vi "message service.vi"(8 "error in":errorcluster, 10 "response queue":T1, 11 "command queue":T1) -> (0 "error out":errorcluster)   [LabVIEW 2013, in "TBD execution service.lvlib"]
doc: "This VI contains a queued message handler process with an associated message API that allows a user to load up a configuration file, launch the configuration, and communicate with the engines contained in that configuration. \n\nThis process can be useful when you want to support the control of this target by one or more connected hosts. It also allows users to change configuration files without rebooting the target."
uses:
  TBD execution service.lvlib
  <vilib>/NI/AMC/Message Queue.ctl
  <vilib>/NI/AMC/Message.ctl
  <vilib>/NI/Tools/Keyed Array/KeyedArray.ctl
  <vilib>/NI/Configuration Framework/class discovery singleton/class discovery singleton methods.ctl
  SubVIs/configuration elements.ctl
  <vilib>/NI/Tag Bus Data Framework/Framework Configuration Classes/platypus configuration/engines cluster.ctl
  <vilib>/NI/Module Execution Interface/Engine Configuration/engine configuration.lvclass
  <vilib>/NI/Tag Bus Module Framework/module configuration/TBM module configuration.lvclass
  <vilib>/NI/Module Execution Interface/Engine Runtime/Engine Runtime Interface.lvclass
  <vilib>/NI/Tag Bus Module Framework/runtime/TBM module execution interface.lvclass
  <vilib>/NI/Tag Bus Data Framework/Framework Configuration Classes/target runtime/PL_Target Runtime.lvclass
  SubVIs/engine status data.ctl
  <vilib>/NI/Module Execution Interface/Engine Runtime/Execution States.ctl
  <vilib>/NI/Module Execution Interface/Engine Runtime/Fault.ctl
  <vilib>/NI/Tag Bus Module Framework/runtime/error classification.ctl
  <vilib>/NI/AMC/Read Termination Message.vi
  <vilib>/NI/AMC/Create Single Message.vi
  <vilib>/NI/AMC/Globals.vi
  <vilib>/NI/Configuration Framework/class discovery singleton/class discovery singleton.lvlib
  <vilib>/NI/AMC/AMC.lvlib
  <vilib>/NI/Tag Bus Module Framework/FPGA manager/methods.ctl
  <vilib>/NI/Tag Bus Module Framework/FPGA manager/FPGA manager.lvlib
  <vilib>/userdefined/High Color/nirio_resource_hc.ctl
  <vilib>/rvi/interface/nirviOpenFPGA/nirviOpenFPGA.xnode
  <vilib>/NI/Tag Bus Data Framework/Framework Configuration Classes/platypus configuration/PLConfigurationSerializer.lvlib
  <vilib>/NI/Configuration Framework/tree serializer/NISE_CEF_TreeSerializer.lvlib
  <vilib>/NI/Tag Bus Data Framework/Framework Configuration Classes/flattened data interface/PL_Serialization Interface.lvlib
  <vilib>/NI/Tools/Keyed Array/Tools_KeyedArray.lvlib
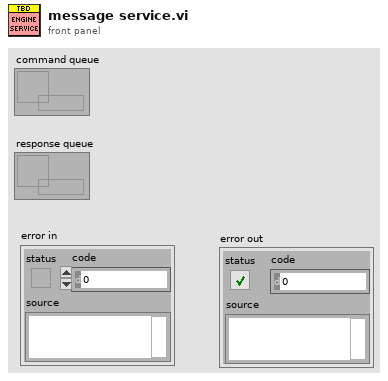
[diagram p1: front panel]
types:
  T1 = typedef "AMC.lvlib/Message Queue.ctl" = refnum<queue>
  T2 = typedef "class discovery singleton.lvlib/class discovery singleton methods.ctl" = enum16{"add search paths", "load class by name", "list available classes", "get class path"}
  T3 = typedef "nirio_resource_hc.ctl" = tag
  T4 = typedef "FPGA manager.lvlib/methods.ctl" = enum16{"initialize bitfile", "cache bitfile", "locate bitfile", "close bitfile"}
  T5 = typedef "TBD execution service.lvlib/configuration elements.ctl" = cluster{"Name":string, "opened?":bool, "configuration":T6, "engine":refnum<class "Engine Runtime Interface.lvclass">, "modules":refnum<class "TBM module execution interface.lvclass">[]}
  T6 = typedef "PLConfigurationSerializer.lvlib/engines cluster.ctl" = cluster{"engine configuration":refnum<class "engine configuration.lvclass">, "modules":refnum<class "TBM module configuration.lvclass">[]}
  T7 = typedef "TBD execution service.lvlib/engine status data.ctl" = cluster{"Name":string, "Engine State":T8, "Faults":T9[], "Engine Error":errorcluster}
  T8 = typedef "Engine Runtime Interface.lvclass/Execution States.ctl" = enum16{"Init", "Pre-Operational", "Safe-Operational", "Operational", "Stopped"}
  T9 = typedef "Engine Runtime Interface.lvclass/Fault.ctl" = cluster{"code":i32, "error classification":T10, "Source GUID":string, "first reported time":timestamp, "number reported":u32, "last reported time":timestamp}
  T10 = typedef "TBM module execution interface.lvclass/error classification.ctl" = enum16{"unknown", "none", "trivial", "recoverable", "critical"}
  T11 = typedef "TBD execution service.lvlib/command commands to rtexe process.ctl" = enum16{"Initialize", "Add Search Paths", "Load from File", "Unload File", "Open All Engines", "Open Single Engine", "Initialize All Engines", "Initialize Single Engine", "Start All", "Start Single", "Pause All", "Pause Single", "Stop All", "Stop Single", "Close All", "Close Single", "Set Safe State All", "Set Safe State Single", "Get Status", "Exit", "Error", "Load Bitfile", "Unload Bitfile", "Clear Faults Single", "Clear Faults All"}
  T12 = typedef "NISE_CEF_TreeSerializer.lvlib/base file format.ctl" = cluster{"version":string, "data":string}
  T13 = typedef "NISE_CEF_TreeSerializer.lvlib/flat hierarchy.ctl" = cluster{"hierarchy structure":T14, "instance data":T16[]}
  T14 = typedef "NISE_CEF_TreeSerializer.lvlib/full hierarchy.ctl" = cluster{"root":string, "hierarchy":T15[]}
  T15 = typedef "NISE_CEF_TreeSerializer.lvlib/hierarchy element.ctl" = cluster{"current node":string, "children":string[]}
  T16 = typedef "NISE_CEF_TreeSerializer.lvlib/instance data.ctl" = cluster{"ID":string, "Alias":string, "class":string, "version":string, "data":string}
  T17 = typedef "PLConfigurationSerializer.lvlib/targets cluster.ctl" = cluster{"Target Configuration":refnum<class "PL_Target Configuration.lvclass">, "engines":T6[]}
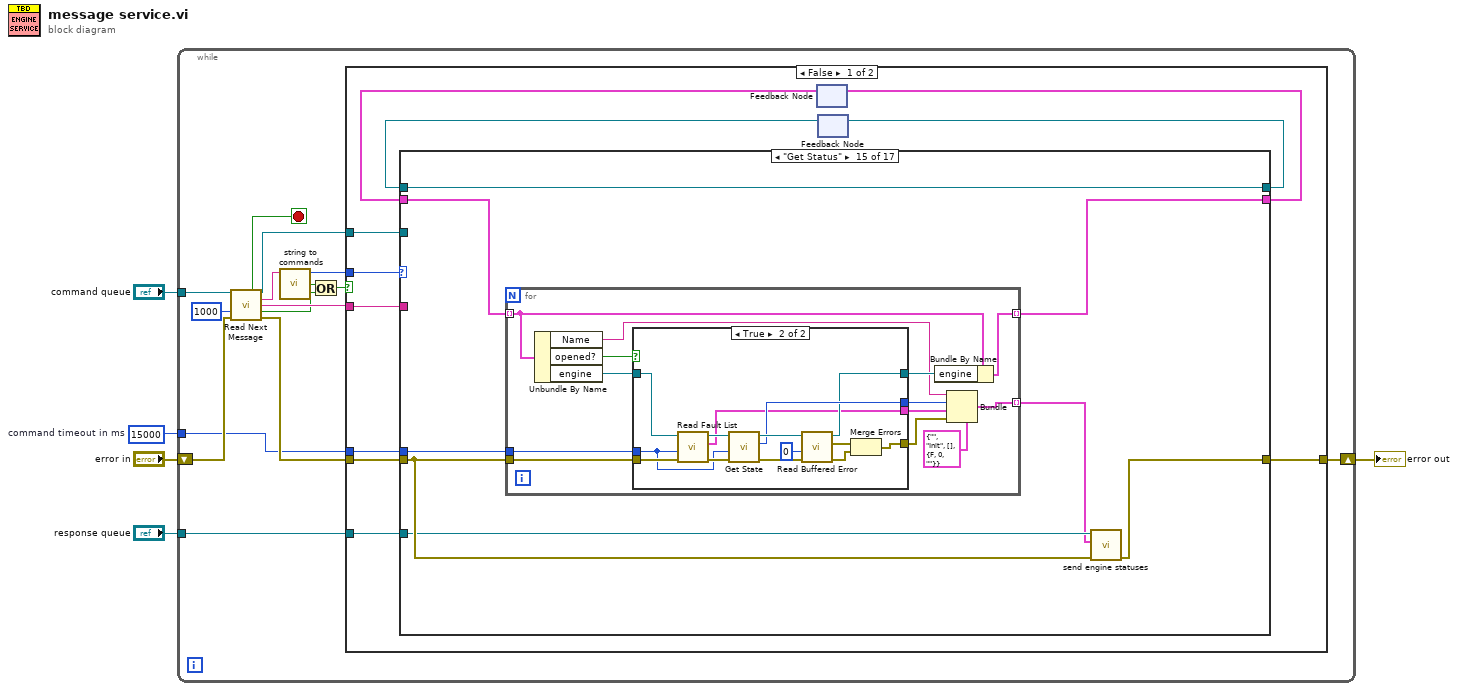
[diagram p0: block diagram]
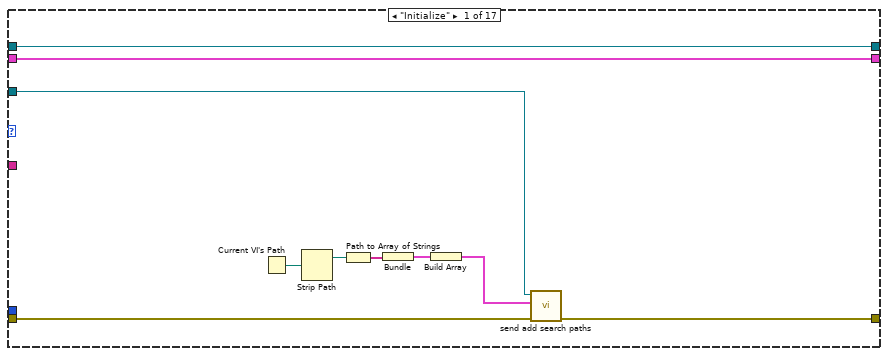
[diagram p2: hidden frame]
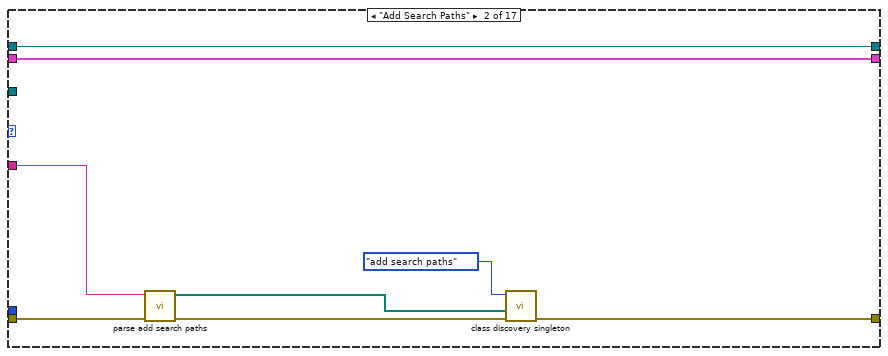
[diagram p3: hidden frame]
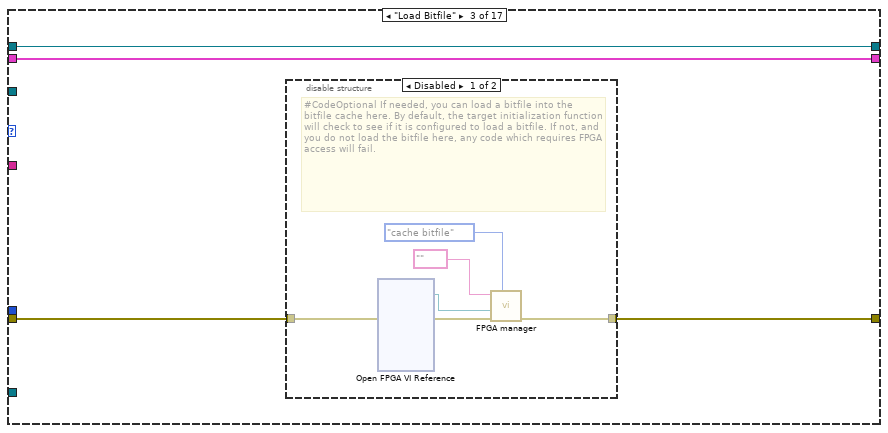
[diagram p4: hidden frame]
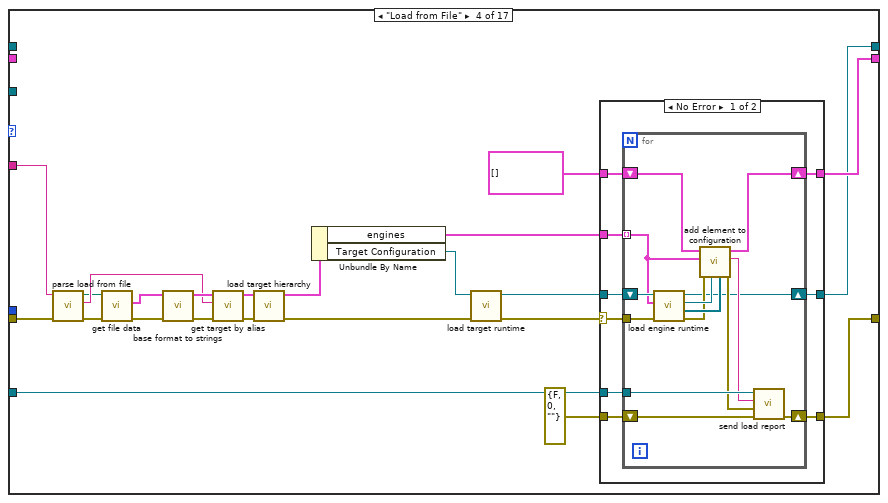
[diagram p6: hidden frame]
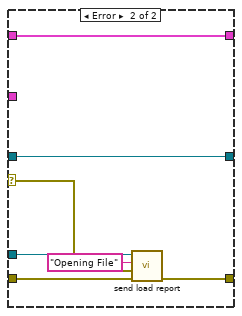
[diagram p7: hidden frame]
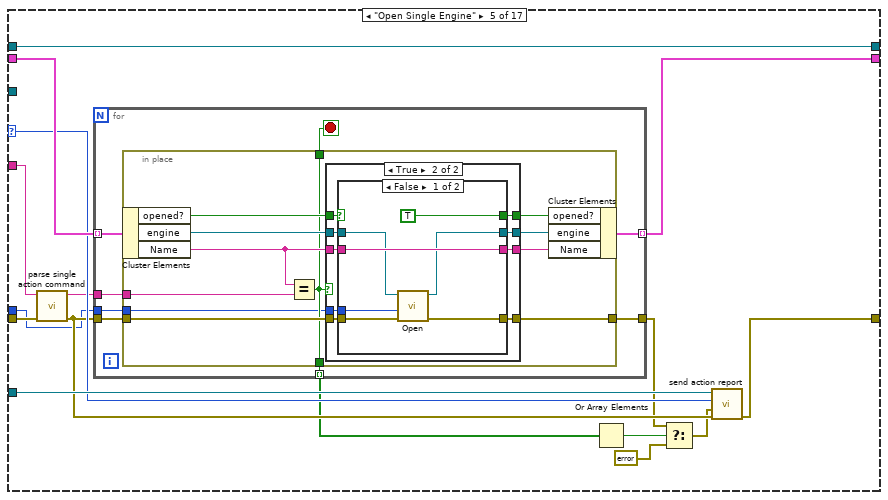
[diagram p8: hidden frame]
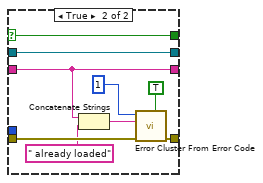
[diagram p10: hidden frame]
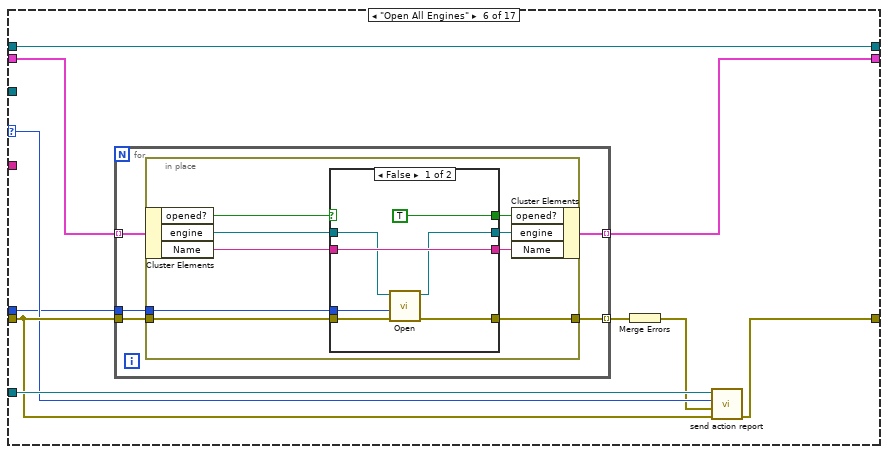
[diagram p11: hidden frame]
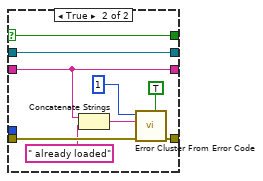
[diagram p12: hidden frame]
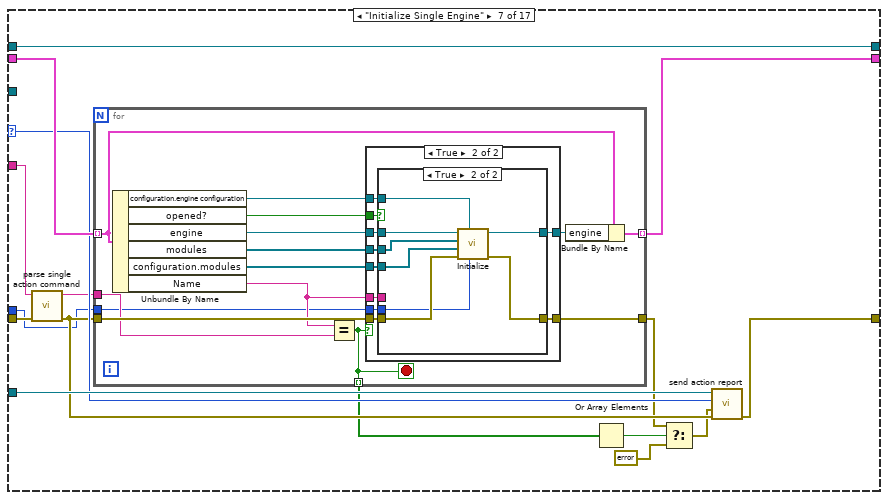
[diagram p13: hidden frame]
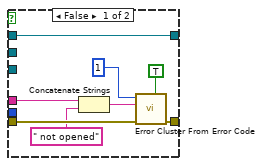
[diagram p15: hidden frame]
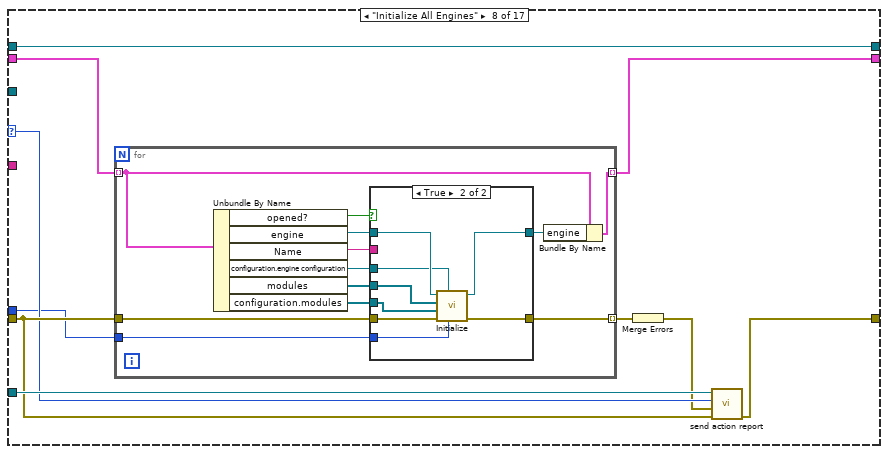
[diagram p16: hidden frame]
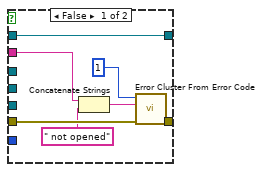
[diagram p17: hidden frame]
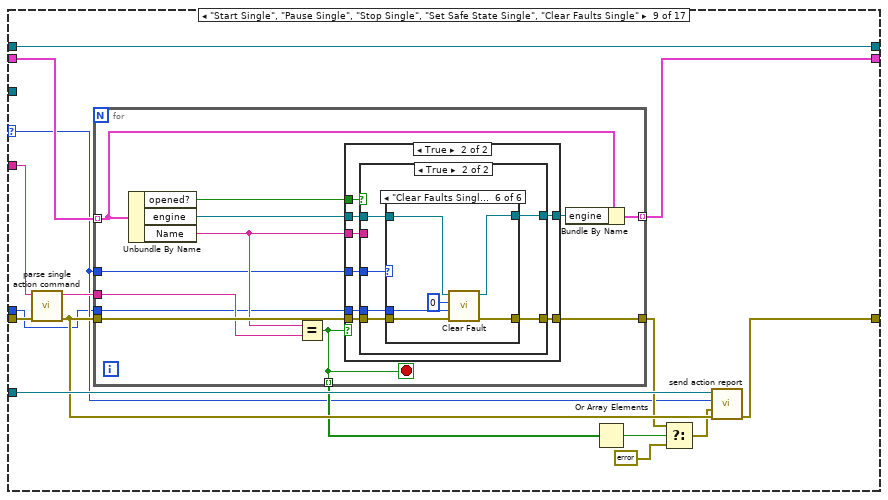
[diagram p18: hidden frame]
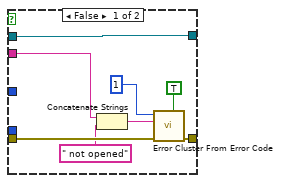
[diagram p20: hidden frame]
diagram:
  w1 = 15000  # command timeout in ms
  n1 = while {
    tunnel: "command queue" -> [w18]
    shift-right: [w20] -> w2
    shift-left: "error in" -> [w15]
    tunnel: "response queue" -> [w19]
    tunnel: w1 -> [w6]
    stop <- w17 stop-if-true
    n2 = call <vilib>:"Read Next Message.vi"("message queue in"=w18, "timeout (1 ms)"=1000, "error in"=w15) -> ("exit process?"=w17:bool, "message queue out"=w7:T1, "message name"=w12:string, "message value"=w16:string, "timed out?"=w10:bool, "error out"=w14:errorcluster)  [unwired: 5 in, 2 out]
    n3 = call "string to commands.vi"("command string"=w12) -> ("invalid"=w11:bool, "commands"=w8:T11)  [unwired: 9 in]
    n4 = Or(x=w11, y=w10) -> (x .or. y?=w9:bool)
    n5 = case shown="False" w9 {
      tunnel: w16 -> [w31 _]
      tunnel: [w30 w654] -> w20
      tunnel: w19 -> [w29 _]
      tunnel: w14 -> [w28 w654]
      tunnel: w8 -> [w27 _]
      tunnel: w7 -> [w26 _]
      tunnel: w6 -> [w21 _]
      frame False {
        n6 = feedback #1() -> (w24:T5[])  [unwired: 1 in]
        n7 = feedback #2() -> (w22:refnum<class "PL_Target Runtime.lvclass">)  [unwired: 1 in]
        n8 = case shown="\"Get Status\"" w27 {
          selector: w27 -> [_ _ _ _ w125 w181 w229 w279 w315 w398 w471 w526 _ _ _ _ w623]
          tunnel: w31 -> [_ w43 _ w83 w122 _ w226 _ w322 _ w468 _ _ _ _ _ _]
          tunnel: [w41 w49 w53 w81 w128 w186 w232 w284 w327 w404 w474 w531 w565 w569 w581 w617 w628] -> w25
          tunnel: w24 -> [w41 w49 w53 _ w129 w187 w233 w285 w328 w405 w475 w532 w565 w569 w582 w617 w629]
          tunnel: [w39 w47 w51 w80 w126 w183 w230 w281 w325 w401 w472 w528 w562 w567 w579 w614 w626] -> w30
          tunnel: w28 -> [w40 w46 w52 w82 w124 w184 w228 w282 w324 w402 w470 w529 w563 w568 w580 w615 w625]
          tunnel: w29 -> [_ _ _ w79 w127 w185 w231 w283 w326 w403 w473 w530 _ _ w578 w613 w624]
          tunnel: w26 -> [w38 _ _ _ _ _ _ _ _ _ _ _ _ _ _ _ _]
          tunnel: [w32 w42 w50 w63 w115 w179 w219 w277 w314 w397 w461 w524 _ w566 w576 w612 w622] -> w23
          tunnel: w22 -> [w32 w42 w50 _ w115 w179 w219 w277 w314 w397 w461 w524 w564 w566 w576 w612 w622]
          tunnel: w21 -> [_ _ _ _ w114 w178 w218 w276 w313 w396 w460 w523 _ _ w575 _ w621]
          frame "Initialize" {
            n9 = Current VI's Path() -> (path=w37:path)
            n10 = Strip Path(path=w37) -> (stripped path=w36:path)  [unwired: 1 out]
            n11 = Path to Array of Strings(0:w36) -> (2:w35:string[])  [unwired: 1 out]
            n12 = Bundle("array of strings"=w35) -> (w34:cluster{"array of strings":string[]})  [unwired: 1 in]
            n13 = Build Array(w34) -> (w33:cluster{"array of strings":string[]}[])
            n14 = call "send add search paths.vi"("error in"=w40, "search paths"=w33, "message queue in"=w38) -> ("error out"=w39:errorcluster)  [unwired: 7 in, 1 out]
          }
          frame "Add Search Paths" {
            n15 = call "parse add search paths.vi"("error in"=w46, "message data"=w43) -> ("error out"=w45:errorcluster, "paths"=w44:path[])  [unwired: 8 in]
            n16 = call <vilib>:"class discovery singleton.vi"("error in"=w45, "Plugin Search Paths"=w44, "method"=class_discovery_singleton_methods."add search paths") -> ("error out"=w47:errorcluster)  [unwired: 5 in, 3 out]
          }
          frame "Load Bitfile" {
            n17 = disable-structure shown="Disabled" {
              disable-tunnel: [w55 w60] -> w51
              disable-tunnel: w52 -> [w54 w60]
              frame Disabled {
                # "#CodeOptional If needed, you can load a bitfile into the bitfile cache here. By default, the target initialization function will check to see if it is configured to load a bitfile. If not, and you do not load the bitfile here, any code which requires FPGA access will fail."
                n18 = xnode "Open FPGA VI Reference"("error in"=w54) -> ("FPGA VI Reference Out"=w58:refnum<k20>, "error out"=w59:errorcluster)  [unwired: 1 in]
                n19 = call <vilib>:"FPGA manager.vi"("action"=methods."cache bitfile", "error in"=w59, "bitfile to cache"=w58, "RIO resource"=T3 "") -> ("error out"=w55:errorcluster)  [unwired: 5 in, 2 out]
              }
              frame Enabled {
              }
            }
          }
          frame "Load from File" {
            n20 = call "parse load from file.vi"("error in"=w82, "message data"=w83) -> ("error out"=w61:errorcluster, "target alias"=w64:string, "path"=w62:path)  [unwired: 7 in]
            n21 = call <vilib>:"get file data.vi"("error in"=w61, "Path"=w62) -> ("error out"=w71:errorcluster, "format"=w72:T12)  [unwired: 8 in]
            n22 = call <vilib>:"base format to strings.vi"("error in"=w71, "format"=w72) -> ("error out"=w66:errorcluster, "data"=w68:T13)  [unwired: 8 in]
            n23 = call <vilib>:"get target by alias.vi"("error in"=w66, "alias"=w64, "system hierarchy"=w68) -> ("error out"=w65:errorcluster, "target hierarchy"=w67:T13)  [unwired: 7 in]
            n24 = call <vilib>:"load target hierarchy.vi"("error in"=w65, "target hierarchy"=w67) -> ("error out"=w69:errorcluster, "targets cluster out"=w70:T17)  [unwired: 8 in]
            n25 = Unbundle By Name(w70) -> ("engines"=w77:T6[], "Target Configuration"=w78:refnum<class "PL_Target Configuration.lvclass">)
            n26 = call <vilib>:"load target runtime.vi"("error in"=w69, "target configuration"=w78) -> ("error out"=w73:errorcluster, "target runtime"=w76:refnum<class "PL_Target Runtime.lvclass">)  [unwired: 8 in]
            n27 = case shown="No Error" w73 {
              selector: w73 -> [w85 w112]
              tunnel: [w92 w113] -> w81
              tunnel: [w91 w110] -> w80
              tunnel: w79 -> [w90 w109]
              tunnel: w77 -> [w89 _]
              tunnel: w76 -> [w88 w107]
              tunnel: errorcluster {"status"=FALSE, "code"=0, "source"=""} ("error out") -> [w87 w111]
              tunnel: T5[] [] ("Configuration out") -> [w86 w113]
              tunnel: [w84 w107] -> w63
              frame No Error {
                n28 = for {
                  shift-right: [w106] -> w92
                  shift-left: w86 -> [w105]
                  shift-right: [w103] -> w91
                  shift-left: w87 -> [w100]
                  tunnel: w90 -> [w104]
                  tunnel: w89 -> [w93] mode=indexing
                  shift-right: [w94] -> w84
                  shift-left: w88 -> [w99]
                  tunnel: w85 -> [w98]
                  n29 = call <vilib>:"load engine runtime.vi"("error in"=w98, "engine configuration in"=w93, "Target Runtime in"=w99) -> ("error out"=w95:errorcluster, "Module Runtime Objects"=w96:refnum<class "TBM module execution interface.lvclass">[], "Engine Runtime Object"=w97:refnum<class "Engine Runtime Interface.lvclass">, "Target Runtime out"=w94:refnum<class "PL_Target Runtime.lvclass">)  [unwired: 5 in]
                  n30 = call "add element to configuration.vi"("Module Runtime Objects"=w96, "Engine Runtime Object"=w97, "error in"=w95, "engine configuration in"=w93, "Configuration in"=w105) -> ("error out"=w101:errorcluster, "engine loaded"=w102:string, "Configuration out"=w106:T5[])  [unwired: 4 in]
                  n31 = call "send load report.vi"("error in"=w100, "load error"=w101, "engine loaded"=w102, "message queue in"=w104) -> ("error out"=w103:errorcluster)  [unwired: 6 in, 1 out]
                }
              }
              frame Error {
                n32 = call "send load report.vi"("error in"=w111, "load error"=w112, "engine loaded"="Opening File", "message queue in"=w109) -> ("error out"=w110:errorcluster)  [unwired: 6 in, 1 out]
              }
            }
          }
          frame "Open Single Engine" {
            n33 = call "parse single action command.vi"("error in"=w124, "message data"=w122) -> ("error out"=w123:errorcluster, "engine name"=w121:string)  [unwired: 8 in]
            n34 = for {
              tunnel: w129 -> [w137] mode=indexing
              tunnel: [w136] -> w128 mode=indexing
              tunnel: w121 -> [w133]
              tunnel: [w132] -> w120 mode=indexing
              tunnel: w123 -> [w135]
              tunnel: [w134] -> w118
              tunnel: w114 -> [w130]
              stop <- w131 stop-if-true
              n35 = in-place {
                in-place-border: w135 -> [w145]
                in-place-border: [w144] -> w134
                in-place-border: w133 -> [w141]
                in-place-border: [w139] -> w132
                in-place-border: [w139] -> w131
                in-place-border: w130 -> [w138]
                n36 = in-place-cluster #3(w137) -> ("opened?"=w148:bool, "engine"=w147:refnum<class "Engine Runtime Interface.lvclass">, "Name"=w140:string)
                n37 = Equal?(x=w140, y=w141) -> (x = y?=w139:bool)
                n38 = case shown="True" w139 {
                  tunnel: w148 -> [w152 w161]
                  tunnel: w147 -> [w151 w160]
                  tunnel: [w151 w159] -> w146
                  tunnel: w145 -> [w149 w158]
                  tunnel: [w149 w157] -> w144
                  tunnel: [w150 w156] -> w143
                  tunnel: [w152 w155] -> w142
                  tunnel: w140 -> [w150 w154]
                  tunnel: w138 -> [_ w153]
                  frame False {
                  }
                  frame True {
                    n39 = case shown="False" w161 {
                      selector: w161 -> [_ w169]
                      tunnel: w160 -> [w165 w177]
                      tunnel: [w164 w177] -> w159
                      tunnel: w158 -> [w168 w176]
                      tunnel: [w167 w175] -> w157
                      tunnel: w154 -> [w166 w170]
                      tunnel: [w166 w170] -> w156
                      tunnel: [TRUE ("opened?") w169] -> w155
                      tunnel: w153 -> [w162 _]
                      frame False {
                        n40 = call-dynamic "Open.vi"("error in"=w168, "timeout (-1)"=w162, "Engine Runtime Interface in"=w165) -> ("error out"=w167:errorcluster, "Engine Runtime Interface out"=w164:refnum<class "Engine Runtime Interface.lvclass">)  [unwired: 7 in]
                      }
                      frame True {
                        n41 = Concatenate Strings(w170, " already loaded" ("string")) -> (w172:string)
                        n42 = call <vilib>:"Error Cluster From Error Code.vi"("is warning? (False)"=TRUE, "error in (no error)"=w176, "error message (\"\")"=w172, "error code (0)"=1) -> ("error out"=w175:errorcluster)  [unwired: 5 in]
                      }
                    }
                  }
                }
                n43 = in-place-cluster #3("opened?"=w142, "engine"=w146, "Name"=w143) -> (w136:T5)
              }
            }
            n44 = Or Array Elements(Boolean array=w120) -> (logical OR=w119:bool)
            n45 = Select(t=w118, s=w119, f=errorcluster {"status"=TRUE, "code"=1, "source"="Not found"}) -> (s? t:f=w117:errorcluster)
            n46 = call "send action report.vi"("error in"=w123, "command error"=w117, "commands"=w125, "message queue in"=w127) -> ("error out"=w126:errorcluster)  [unwired: 6 in, 1 out]
          }
          frame "Open All Engines" {
            n47 = for {
              tunnel: w187 -> [w192] mode=indexing
              tunnel: [w191] -> w186 mode=indexing
              tunnel: w184 -> [w190]
              tunnel: [w189] -> w182 mode=indexing
              tunnel: w178 -> [w188]
              n48 = in-place {
                in-place-border: w190 -> [w198]
                in-place-border: [w197] -> w189
                in-place-border: w188 -> [w193]
                n49 = in-place-cluster #4(w192) -> ("opened?"=w201:bool, "engine"=w200:refnum<class "Engine Runtime Interface.lvclass">, "Name"=w196:string)
                n50 = case shown="False" w201 {
                  selector: w201 -> [_ w209]
                  tunnel: w200 -> [w205 w217]
                  tunnel: [w204 w217] -> w199
                  tunnel: w198 -> [w208 w216]
                  tunnel: [w207 w215] -> w197
                  tunnel: w196 -> [w206 w210]
                  tunnel: [w206 w210] -> w195
                  tunnel: [TRUE ("opened?") w209] -> w194
                  tunnel: w193 -> [w202 _]
                  frame False {
                    n51 = call-dynamic "Open.vi"("error in"=w208, "timeout (-1)"=w202, "Engine Runtime Interface in"=w205) -> ("error out"=w207:errorcluster, "Engine Runtime Interface out"=w204:refnum<class "Engine Runtime Interface.lvclass">)  [unwired: 7 in]
                  }
                  frame True {
                    n52 = Concatenate Strings(w210, " already loaded" ("string")) -> (w212:string)
                    n53 = call <vilib>:"Error Cluster From Error Code.vi"("is warning? (False)"=TRUE, "error in (no error)"=w216, "error message (\"\")"=w212, "error code (0)"=1) -> ("error out"=w215:errorcluster)  [unwired: 5 in]
                  }
                }
                n54 = in-place-cluster #4("opened?"=w194, "engine"=w199, "Name"=w195) -> (w191:T5)
              }
            }
            n55 = Merge Errors(w182) -> (w180:errorcluster)
            n56 = call "send action report.vi"("error in"=w184, "command error"=w180, "commands"=w181, "message queue in"=w185) -> ("error out"=w183:errorcluster)  [unwired: 6 in, 1 out]
          }
          frame "Initialize Single Engine" {
            n57 = call "parse single action command.vi"("error in"=w228, "message data"=w226) -> ("error out"=w227:errorcluster, "engine name"=w225:string)  [unwired: 8 in]
            n58 = for {
              tunnel: w233 -> [w247] mode=indexing
              tunnel: [w246] -> w232 mode=indexing
              tunnel: w225 -> [w243]
              tunnel: [w242] -> w224 mode=indexing
              tunnel: w227 -> [w245]
              tunnel: [w244] -> w222
              tunnel: w218 -> [w234]
              stop <- w242 stop-if-true
              n59 = Unbundle By Name(w247) -> ("configuration.engine configuration"=w235:refnum<class "engine configuration.lvclass">, "opened?"=w241:bool, "engine"=w240:refnum<class "Engine Runtime Interface.lvclass">, "modules"=w236:refnum<class "TBM module execution interface.lvclass">[], "configuration.modules"=w237:refnum<class "TBM module configuration.lvclass">[], "Name"=w238:string)
              n60 = Equal?(x=w238, y=w243) -> (x = y?=w242:bool)
              n61 = case shown="True" w242 {
                tunnel: w241 -> [_ w259]
                tunnel: w240 -> [w249 w258]
                tunnel: [w249 w257] -> w239
                tunnel: w245 -> [w248 w256]
                tunnel: [w248 w255] -> w244
                tunnel: w238 -> [_ w254]
                tunnel: w237 -> [_ w253]
                tunnel: w236 -> [_ w252]
                tunnel: w235 -> [_ w251]
                tunnel: w234 -> [_ w250]
                frame False {
                }
                frame True {
                  n62 = case shown="True" w259 {
                    tunnel: w258 -> [w267 w274]
                    tunnel: [w267 w273] -> w257
                    tunnel: w256 -> [w266 w275]
                    tunnel: [w265 w272] -> w255
                    tunnel: w254 -> [w260 _]
                    tunnel: w253 -> [_ w271]
                    tunnel: w252 -> [_ w270]
                    tunnel: w251 -> [_ w269]
                    tunnel: w250 -> [_ w268]
                    frame False {
                      n63 = Concatenate Strings(w260, " not opened" ("string")) -> (w262:string)
                      n64 = call <vilib>:"Error Cluster From Error Code.vi"("is warning? (False)"=TRUE, "error in (no error)"=w266, "error message (\"\")"=w262, "error code (0)"=1) -> ("error out"=w265:errorcluster)  [unwired: 5 in]
                    }
                    frame True {
                      n65 = call-dynamic "Initialize.vi"("timeout in ms"=w268, "Engine Configuration"=w269, "error in"=w275, "module Configurations"=w271, "modules"=w270, "Engine Runtime Interface in"=w274) -> ("error out"=w272:errorcluster, "Engine Runtime Interface out"=w273:refnum<class "Engine Runtime Interface.lvclass">)  [unwired: 4 in]
                    }
                  }
                }
              }
              n66 = Bundle By Name(cluster=w247, "engine"=w239) -> (w246:T5)
            }
            n67 = Or Array Elements(Boolean array=w224) -> (logical OR=w223:bool)
            n68 = Select(t=w222, s=w223, f=errorcluster {"status"=TRUE, "code"=1, "source"="Not found"}) -> (s? t:f=w221:errorcluster)
            n69 = call "send action report.vi"("error in"=w227, "command error"=w221, "commands"=w229, "message queue in"=w231) -> ("error out"=w230:errorcluster)  [unwired: 6 in, 1 out]
          }
          frame "Initialize All Engines" {
            n70 = for {
              tunnel: w285 -> [w297] mode=indexing
              tunnel: [w296] -> w284 mode=indexing
              tunnel: w282 -> [w295]
              tunnel: [w294] -> w280 mode=indexing
              tunnel: w276 -> [w286]
              n71 = Unbundle By Name(w297) -> ("opened?"=w293:bool, "engine"=w292:refnum<class "Engine Runtime Interface.lvclass">, "Name"=w290:string, "configuration.engine configuration"=w289:refnum<class "engine configuration.lvclass">, "modules"=w288:refnum<class "TBM module execution interface.lvclass">[], "configuration.modules"=w287:refnum<class "TBM module configuration.lvclass">[])
              n72 = case shown="True" w293 {
                tunnel: w292 -> [w304 w309]
                tunnel: [w304 w310] -> w291
                tunnel: w295 -> [w303 w311]
                tunnel: [w302 w312] -> w294
                tunnel: w290 -> [w298 _]
                tunnel: w289 -> [_ w308]
                tunnel: w288 -> [_ w307]
                tunnel: w287 -> [_ w306]
                tunnel: w286 -> [_ w305]
                frame False {
                  n73 = Concatenate Strings(w298, " not opened" ("string")) -> (w300:string)
                  n74 = call <vilib>:"Error Cluster From Error Code.vi"("error in (no error)"=w303, "error message (\"\")"=w300, "error code (0)"=1) -> ("error out"=w302:errorcluster)  [unwired: 6 in]
                }
                frame True {
                  n75 = call-dynamic "Initialize.vi"("timeout in ms"=w305, "Engine Configuration"=w308, "error in"=w311, "module Configurations"=w306, "modules"=w307, "Engine Runtime Interface in"=w309) -> ("error out"=w312:errorcluster, "Engine Runtime Interface out"=w310:refnum<class "Engine Runtime Interface.lvclass">)  [unwired: 4 in]
                }
              }
              n76 = Bundle By Name(cluster=w297, "engine"=w291) -> (w296:T5)
            }
            n77 = Merge Errors(w280) -> (w278:errorcluster)
            n78 = call "send action report.vi"("error in"=w282, "command error"=w278, "commands"=w279, "message queue in"=w283) -> ("error out"=w281:errorcluster)  [unwired: 6 in, 1 out]
          }
          frame "Start Single", "Pause Single", "Stop Single", "Set Safe State Single", "Clear Faults Single" {
            n79 = call "parse single action command.vi"("error in"=w324, "message data"=w322) -> ("error out"=w323:errorcluster, "engine name"=w321:string)  [unwired: 8 in]
            n80 = for {
              tunnel: w328 -> [w340] mode=indexing
              tunnel: [w339] -> w327 mode=indexing
              tunnel: w321 -> [w336]
              tunnel: [w335] -> w320 mode=indexing
              tunnel: w323 -> [w338]
              tunnel: [w337] -> w318
              tunnel: w315 -> [w330]
              tunnel: w313 -> [w329]
              stop <- w335 stop-if-true
              n81 = Unbundle By Name(w340) -> ("opened?"=w334:bool, "engine"=w333:refnum<class "Engine Runtime Interface.lvclass">, "Name"=w331:string)
              n82 = Equal?(x=w331, y=w336) -> (x = y?=w335:bool)
              n83 = case shown="True" w335 {
                tunnel: w334 -> [_ w350]
                tunnel: w333 -> [w342 w349]
                tunnel: [w342 w348] -> w332
                tunnel: w338 -> [w341 w347]
                tunnel: [w341 w346] -> w337
                tunnel: w331 -> [_ w345]
                tunnel: w330 -> [_ w344]
                tunnel: w329 -> [_ w343]
                frame False {
                }
                frame True {
                  n84 = case shown="True" w350 {
                    tunnel: w349 -> [w358 w362]
                    tunnel: [w358 w363] -> w348
                    tunnel: w347 -> [w357 w361]
                    tunnel: [w356 w364] -> w346
                    tunnel: w345 -> [w351 _]
                    tunnel: w344 -> [_ w360]
                    tunnel: w343 -> [_ w359]
                    frame False {
                      n85 = Concatenate Strings(w351, " not opened" ("string")) -> (w353:string)
                      n86 = call <vilib>:"Error Cluster From Error Code.vi"("is warning? (False)"=TRUE, "error in (no error)"=w357, "error message (\"\")"=w353, "error code (0)"=1) -> ("error out"=w356:errorcluster)  [unwired: 5 in]
                    }
                    frame True {
                      n87 = case shown="\"Clear Faults Single\"" w360 {
                        tunnel: w361 -> [w367 w374 w379 w384 w389 w393]
                        tunnel: [w368 w373 w378 w383 w388 w392] -> w364
                        tunnel: [w369 w372 w377 w382 w386 w390] -> w363
                        tunnel: w362 -> [w369 w371 w376 w381 w387 w391]
                        tunnel: w359 -> [_ w370 w375 w380 w385 w394]
                        frame Default {
                          n88 = call <vilib>:"Error Cluster From Error Code.vi"("error in (no error)"=w367, "error message (\"\")"="dev" ("error message (\"\")"), "error code (0)"=42) -> ("error out"=w368:errorcluster)  [unwired: 6 in]
                        }
                        frame "Start Single" {
                          n89 = call-dynamic "Start.vi"("error in"=w374, "timeout (-1)"=w370, "Engine Runtime Interface in"=w371) -> ("error out"=w373:errorcluster, "Engine Runtime Interface out"=w372:refnum<class "Engine Runtime Interface.lvclass">)  [unwired: 7 in]
                        }
                        frame "Pause Single" {
                          n90 = call-dynamic "Pause.vi"("error in"=w379, "timeout (-1)"=w375, "Engine Runtime Interface in"=w376) -> ("error out"=w378:errorcluster, "Engine Runtime Interface out"=w377:refnum<class "Engine Runtime Interface.lvclass">)  [unwired: 7 in]
                        }
                        frame "Set Safe State Single" {
                          n91 = call-dynamic "Set Safe State.vi"("error in"=w384, "timeout (-1)"=w380, "Engine Runtime Interface in"=w381) -> ("error out"=w383:errorcluster, "Engine Runtime Interface out"=w382:refnum<class "Engine Runtime Interface.lvclass">)  [unwired: 7 in]
                        }
                        frame "Stop Single" {
                          n92 = call-dynamic "Stop.vi"("error in"=w389, "timeout (-1)"=w385, "Engine Runtime Interface in"=w387) -> ("error out"=w388:errorcluster, "Engine Runtime Interface out"=w386:refnum<class "Engine Runtime Interface.lvclass">)  [unwired: 7 in]
                        }
                        frame "Clear Faults Single" {
                          n93 = call-dynamic "Clear Fault.vi"("error in"=w393, "timeout (-1)"=w394, "code (0=clear all)"=0, "Engine Runtime Interface in"=w391) -> ("error out"=w392:errorcluster, "Engine Runtime Interface out"=w390:refnum<class "Engine Runtime Interface.lvclass">)  [unwired: 6 in]
                        }
                      }
                    }
                  }
                }
              }
              n94 = Bundle By Name(cluster=w340, "engine"=w332) -> (w339:T5)
            }
            n95 = Or Array Elements(Boolean array=w320) -> (logical OR=w319:bool)
            n96 = Select(t=w318, s=w319, f=errorcluster {"status"=TRUE, "code"=1, "source"="Not found"}) -> (s? t:f=w317:errorcluster)
            n97 = call "send action report.vi"("error in"=w323, "command error"=w317, "commands"=w315, "message queue in"=w326) -> ("error out"=w325:errorcluster)  [unwired: 6 in, 1 out]
          }
          frame "Start All", "Pause All", "Stop All", "Set Safe State All", "Clear Faults All" {
            n98 = for {
              tunnel: w405 -> [w415] mode=indexing
              tunnel: [w414] -> w404 mode=indexing
              tunnel: w402 -> [w413]
              tunnel: [w412] -> w400 mode=indexing
              tunnel: w398 -> [w407]
              tunnel: w396 -> [w406]
              n99 = Unbundle By Name(w415) -> ("opened?"=w411:bool, "engine"=w410:refnum<class "Engine Runtime Interface.lvclass">, "Name"=w408:string)
              n100 = case shown="True" w411 {
                tunnel: w410 -> [w422 w425]
                tunnel: [w422 w426] -> w409
                tunnel: w413 -> [w421 w428]
                tunnel: [w420 w427] -> w412
                tunnel: w408 -> [w416 _]
                tunnel: w407 -> [_ w424]
                tunnel: w406 -> [_ w423]
                frame False {
                  n101 = Concatenate Strings(w416, " not opened" ("string")) -> (w418:string)
                  n102 = call <vilib>:"Error Cluster From Error Code.vi"("error in (no error)"=w421, "error message (\"\")"=w418, "error code (0)"=1) -> ("error out"=w420:errorcluster)  [unwired: 6 in]
                }
                frame True {
                  n103 = case shown="\"Clear Faults All\"" w424 {
                    tunnel: w428 -> [w431 w438 w443 w448 w453 w458]
                    tunnel: [w432 w437 w442 w447 w452 w454] -> w427
                    tunnel: [w433 w436 w441 w445 w451 w455] -> w426
                    tunnel: w425 -> [w433 w435 w440 w446 w450 w456]
                    tunnel: w423 -> [_ w434 w439 w444 w449 w457]
                    frame Default {
                      n104 = call <vilib>:"Error Cluster From Error Code.vi"("error in (no error)"=w431, "error message (\"\")"="dev" ("error message (\"\")"), "error code (0)"=42) -> ("error out"=w432:errorcluster)  [unwired: 6 in]
                    }
                    frame "Start All" {
                      n105 = call-dynamic "Start.vi"("error in"=w438, "timeout (-1)"=w434, "Engine Runtime Interface in"=w435) -> ("error out"=w437:errorcluster, "Engine Runtime Interface out"=w436:refnum<class "Engine Runtime Interface.lvclass">)  [unwired: 7 in]
                    }
                    frame "Pause All" {
                      n106 = call-dynamic "Pause.vi"("error in"=w443, "timeout (-1)"=w439, "Engine Runtime Interface in"=w440) -> ("error out"=w442:errorcluster, "Engine Runtime Interface out"=w441:refnum<class "Engine Runtime Interface.lvclass">)  [unwired: 7 in]
                    }
                    frame "Stop All" {
                      n107 = call-dynamic "Stop.vi"("error in"=w448, "timeout (-1)"=w444, "Engine Runtime Interface in"=w446) -> ("error out"=w447:errorcluster, "Engine Runtime Interface out"=w445:refnum<class "Engine Runtime Interface.lvclass">)  [unwired: 7 in]
                    }
                    frame "Set Safe State All" {
                      n108 = call-dynamic "Set Safe State.vi"("error in"=w453, "timeout (-1)"=w449, "Engine Runtime Interface in"=w450) -> ("error out"=w452:errorcluster, "Engine Runtime Interface out"=w451:refnum<class "Engine Runtime Interface.lvclass">)  [unwired: 7 in]
                    }
                    frame "Clear Faults All" {
                      n109 = call-dynamic "Clear Fault.vi"("error in"=w458, "timeout (-1)"=w457, "code (0=clear all)"=0, "Engine Runtime Interface in"=w456) -> ("error out"=w454:errorcluster, "Engine Runtime Interface out"=w455:refnum<class "Engine Runtime Interface.lvclass">)  [unwired: 6 in]
                    }
                  }
                }
              }
              n110 = Bundle By Name(cluster=w415, "engine"=w409) -> (w414:T5)
            }
            n111 = Merge Errors(w400) -> (w399:errorcluster)
            n112 = call "send action report.vi"("error in"=w402, "command error"=w399, "commands"=w398, "message queue in"=w403) -> ("error out"=w401:errorcluster)  [unwired: 6 in, 1 out]
          }
          frame "Close Single" {
            n113 = call "parse single action command.vi"("error in"=w470, "message data"=w468) -> ("error out"=w469:errorcluster, "engine name"=w467:string)  [unwired: 8 in]
            n114 = for {
              tunnel: w475 -> [w483] mode=indexing
              tunnel: [w482] -> w474 mode=indexing
              tunnel: w467 -> [w479]
              tunnel: [w478] -> w466 mode=indexing
              tunnel: w469 -> [w481]
              tunnel: [w480] -> w464
              tunnel: w460 -> [w476]
              stop <- w477 stop-if-true
              n115 = in-place {
                in-place-border: w481 -> [w491]
                in-place-border: [w490] -> w480
                in-place-border: w479 -> [w487]
                in-place-border: [w485] -> w478
                in-place-border: [w485] -> w477
                in-place-border: w476 -> [w484]
                n116 = in-place-cluster #5(w483) -> ("opened?"=w494:bool, "engine"=w493:refnum<class "Engine Runtime Interface.lvclass">, "Name"=w486:string)
                n117 = Equal?(x=w486, y=w487) -> (x = y?=w485:bool)
                n118 = case shown="True" w485 {
                  tunnel: w494 -> [w498 w507]
                  tunnel: w493 -> [w497 w506]
                  tunnel: [w497 w505] -> w492
                  tunnel: w491 -> [w495 w504]
                  tunnel: [w495 w503] -> w490
                  tunnel: [w496 w502] -> w489
                  tunnel: [w498 w501] -> w488
                  tunnel: w486 -> [w496 w500]
                  tunnel: w484 -> [_ w499]
                  frame False {
                  }
                  frame True {
                    n119 = case shown="False" w507 {
                      selector: w507 -> [w508 _]
                      tunnel: w506 -> [w516 w518]
                      tunnel: [w516 w518] -> w505
                      tunnel: w504 -> [w515 w519]
                      tunnel: [w514 w520] -> w503
                      tunnel: w500 -> [w509 w522]
                      tunnel: [w509 w522] -> w502
                      tunnel: [w508 FALSE ("opened?")] -> w501
                      tunnel: w499 -> [_ w517]
                      frame False {
                        n120 = Concatenate Strings(w509, " not opened" ("string")) -> (w511:string)
                        n121 = call <vilib>:"Error Cluster From Error Code.vi"("is warning? (False)"=TRUE, "error in (no error)"=w515, "error message (\"\")"=w511, "error code (0)"=1) -> ("error out"=w514:errorcluster)  [unwired: 5 in]
                      }
                      frame True {
                        n122 = call-dynamic "Close.vi"("error in"=w519, "timeout (-1)"=w517, "Engine Runtime Interface in"=w518) -> ("error out"=w520:errorcluster)  [unwired: 8 in]
                      }
                    }
                  }
                }
                n123 = in-place-cluster #5("opened?"=w488, "engine"=w492, "Name"=w489) -> (w482:T5)
              }
            }
            n124 = Or Array Elements(Boolean array=w466) -> (logical OR=w465:bool)
            n125 = Select(t=w464, s=w465, f=errorcluster {"status"=TRUE, "code"=1, "source"="Not found"}) -> (s? t:f=w463:errorcluster)
            n126 = call "send action report.vi"("error in"=w469, "command error"=w463, "commands"=w471, "message queue in"=w473) -> ("error out"=w472:errorcluster)  [unwired: 6 in, 1 out]
          }
          frame "Close All" {
            n127 = for {
              tunnel: w532 -> [w537] mode=indexing
              tunnel: [w536] -> w531 mode=indexing
              tunnel: w529 -> [w535]
              tunnel: [w534] -> w527 mode=indexing
              tunnel: w523 -> [w533]
              n128 = in-place {
                in-place-border: w535 -> [w543]
                in-place-border: [w542] -> w534
                in-place-border: w533 -> [w538]
                n129 = in-place-cluster #6(w537) -> ("opened?"=w546:bool, "engine"=w545:refnum<class "Engine Runtime Interface.lvclass">, "Name"=w541:string)
                n130 = case shown="True" w546 {
                  selector: w546 -> [w547 _]
                  tunnel: w545 -> [w555 w557]
                  tunnel: [w555 w557] -> w544
                  tunnel: w543 -> [w554 w559]
                  tunnel: [w553 w558] -> w542
                  tunnel: w541 -> [w548 w561]
                  tunnel: [w548 w561] -> w540
                  tunnel: [w547 FALSE ("opened?")] -> w539
                  tunnel: w538 -> [_ w556]
                  frame False {
                    n131 = Concatenate Strings(w548, " not open" ("string")) -> (w550:string)
                    n132 = call <vilib>:"Error Cluster From Error Code.vi"("is warning? (False)"=TRUE, "error in (no error)"=w554, "error message (\"\")"=w550, "error code (0)"=1) -> ("error out"=w553:errorcluster)  [unwired: 5 in]
                  }
                  frame True {
                    n133 = call-dynamic "Close.vi"("error in"=w559, "timeout (-1)"=w556, "Engine Runtime Interface in"=w557) -> ("error out"=w558:errorcluster)  [unwired: 8 in]
                  }
                }
                n134 = in-place-cluster #6("opened?"=w539, "engine"=w544, "Name"=w540) -> (w536:T5)
              }
            }
            n135 = Merge Errors(w527) -> (w525:errorcluster)
            n136 = call "send action report.vi"("error in"=w529, "command error"=w525, "commands"=w526, "message queue in"=w530) -> ("error out"=w528:errorcluster)  [unwired: 6 in, 1 out]
          }
          frame "Unload File" {
            n137 = call-dynamic "shutdown.vi"("error in"=w563, "Target Runtime in"=w564) -> ("error out"=w562:errorcluster)  [unwired: 9 in]
          }
          frame "Unload Bitfile" {
            n138 = disable-structure shown="Disabled" {
              disable-tunnel: w568 -> [w571 w574]
              disable-tunnel: [w570 w574] -> w567
              frame Disabled {
                # "#CodeOptional If the bitfile is initialized outside the framework, it should be closed outside the framework"
                n139 = call <vilib>:"FPGA manager.vi"("action"=methods."close bitfile", "error in"=w571, "RIO resource"=T3 "") -> ("error out"=w570:errorcluster)  [unwired: 6 in, 2 out]
              }
              frame Enabled {
              }
            }
          }
          frame "Get Status" {
            n140 = for {
              tunnel: w582 -> [w595] mode=indexing
              tunnel: [w594] -> w581 mode=indexing
              tunnel: w580 -> [w593]
              tunnel: [w589] -> w577 mode=indexing
              tunnel: w575 -> [w585]
              n141 = Unbundle By Name(w595) -> ("Name"=w586:string, "opened?"=w592:bool, "engine"=w591:refnum<class "Engine Runtime Interface.lvclass">)
              n142 = case shown="True" w592 {
                tunnel: w591 -> [w597 w604]
                tunnel: [w597 w608] -> w590
                tunnel: w593 -> [_ w603]
                tunnel: [Execution_States."Init" ("Engine State") w609] -> w587
                tunnel: [_ w606] -> w583
                tunnel: [_ w600] -> w584
                tunnel: w585 -> [_ w599]
                frame False {
                }
                frame True {
                  n143 = call-dynamic "Read Fault List.vi"("error in"=w603, "timeout (-1)"=w599, "Engine Runtime Interface in"=w604) -> ("error out"=w602:errorcluster, "faults"=w600:T9[], "Engine Runtime Interface out"=w601:refnum<class "Engine Runtime Interface.lvclass">)  [unwired: 6 in]
                  n144 = call-dynamic "Get State.vi"("error in"=w602, "timeout (-1)"=w599, "Engine Runtime Interface in"=w601) -> ("error out"=w611:errorcluster, "Engine State"=w609:T8, "Engine Runtime Interface out"=w610:refnum<class "Engine Runtime Interface.lvclass">)  [unwired: 6 in]
                  n145 = call-dynamic "Read Buffered Error.vi"("error in"=w611, "timeout in ms (0)"=0, "Engine Runtime Interface in"=w610) -> ("error out"=w605:errorcluster, "Engine Error"=w607:errorcluster, "Engine Runtime Interface out"=w608:refnum<class "Engine Runtime Interface.lvclass">)  [unwired: 6 in]
                  n146 = Merge Errors(w607, w605) -> (w606:errorcluster)
                }
              }
              n147 = Bundle By Name(cluster=w595, "engine"=w590) -> (w594:T5)
              n148 = Bundle(cluster=T7 {"Name"="", "Engine State"=enum."Init", "Faults"=[], "Engine Error"={"status"=FALSE, "code"=0, "source"=""}}, "Name"=w586, "Engine State"=w587, "Faults"=w584, "Engine Error"=w583) -> (w589:T7)
            }
            n149 = call "send engine statuses.vi"("error in"=w580, "statuses"=w577, "message queue in"=w578) -> ("error out"=w579:errorcluster)  [unwired: 7 in, 1 out]
          }
          frame "Error" {
            # "#CodeRecommended Add error handling code here"
            n150 = Unbundle By Name(w615) -> ("code"=w616:i32)
            n151 = case shown="Default" w616 {
              tunnel: w615 -> [w618 _]
              tunnel: [w619 _] -> w614
              tunnel: w613 -> [w620 _]
              frame Default {
                n152 = call "send error message.vi"("error to send"=w618, "message queue in"=w620) -> ("error out"=w619:errorcluster)  [unwired: 8 in, 1 out]
              }
              frame 538255 {
                # "Ignore this timeout error for now."
              }
            }
          }
          frame "Exit" {
            n153 = for {
              tunnel: w629 -> [w634] mode=indexing
              tunnel: [w633] -> w628 mode=indexing
              tunnel: w625 -> [w632]
              tunnel: [w631] -> w627 mode=indexing
              tunnel: w621 -> [w630]
              n154 = in-place {
                in-place-border: w632 -> [w640]
                in-place-border: [w639] -> w631
                in-place-border: w630 -> [w635]
                n155 = in-place-cluster #7(w634) -> ("opened?"=w643:bool, "engine"=w642:refnum<class "Engine Runtime Interface.lvclass">, "Name"=w638:string)
                n156 = case shown="False" w643 {
                  selector: w643 -> [w644 _]
                  tunnel: w642 -> [w647 w649]
                  tunnel: [w647 w649] -> w641
                  tunnel: w640 -> [w646 w651]
                  tunnel: [w646 w650] -> w639
                  tunnel: w638 -> [w645 w653]
                  tunnel: [w645 w653] -> w637
                  tunnel: [w644 FALSE ("opened?")] -> w636
                  tunnel: w635 -> [_ w648]
                  frame False {
                  }
                  frame True {
                    n157 = call-dynamic "Close.vi"("error in"=w651, "timeout (-1)"=w648, "Engine Runtime Interface in"=w649) -> ("error out"=w650:errorcluster)  [unwired: 8 in]
                  }
                }
                n158 = in-place-cluster #7("opened?"=w636, "engine"=w641, "Name"=w637) -> (w633:T5)
              }
            }
            n159 = Merge Errors(w627) -> (w626:errorcluster)
            n160 = call "send action report.vi"("error in"=w625, "command error"=w626, "commands"=w623, "message queue in"=w624) -> ()  [unwired: 6 in, 2 out]
          }
        }
        n161 = feedback-in #1(w25) -> ()
        n162 = feedback-in #2(w23) -> ()
      }
      frame True {
      }
    }
  }
  "error out" <- w2
